vi "conexionDB.vi"() -> ()   [LabVIEW 2016]
uses:
  <vilib>/addons/database/Connection.llb/DB Tools Open Connec (Path).vi
  <vilib>/addons/database/NI_Database_API.lvlib
panel:
  out "data":variant[][](array[variant])
  out "Table Control":string[][](table)
  out "Multicolumn Listbox":i32(listbox)
  out "data 2":string[][](array[string])
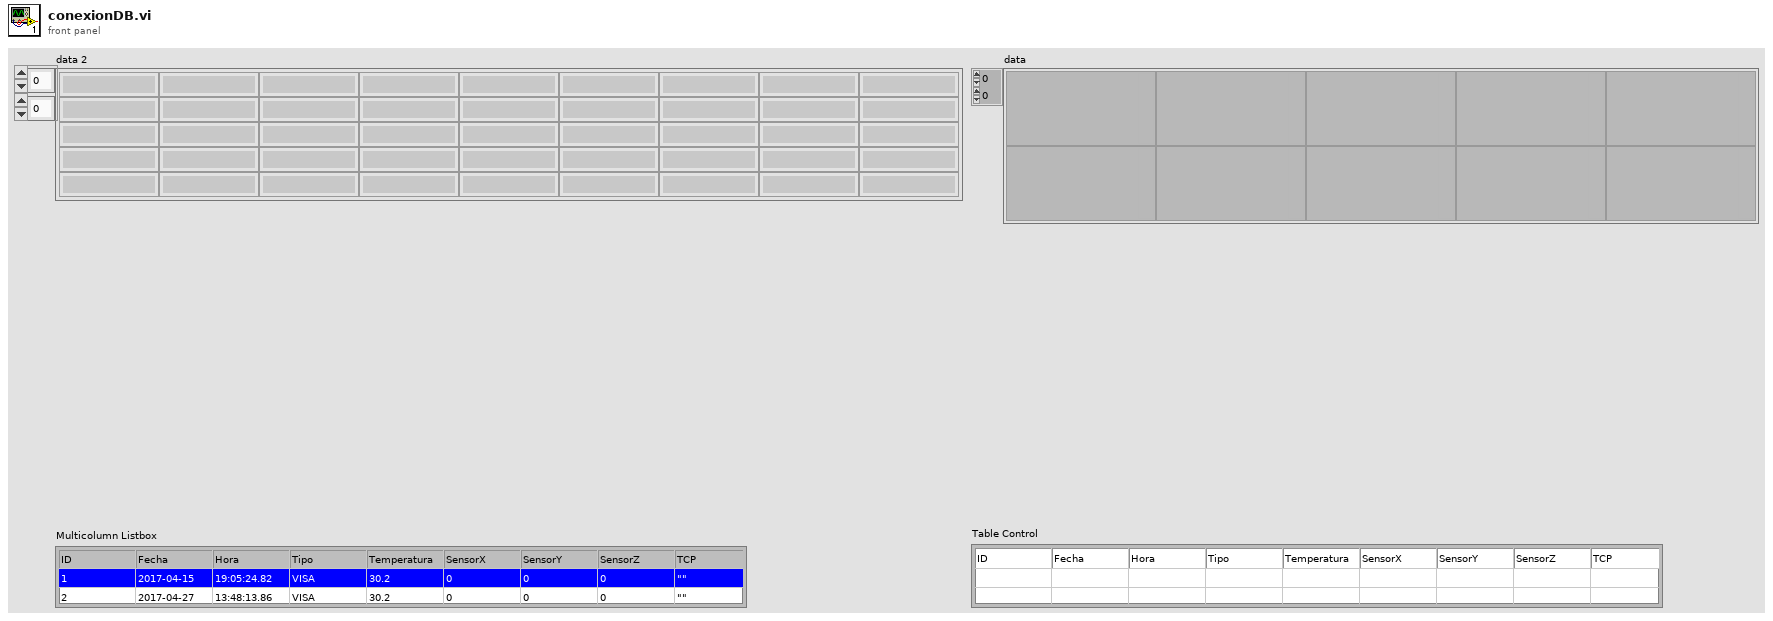
[diagram p1: front panel]
types:
  T1 = typedef "NI_Database_API.lvlib/Conn ObjectReference.ctl" = refnum<k1>
  T2 = cluster{"date/time string":string, "date/time string":string, string, dbl, dbl, dbl, dbl, string}
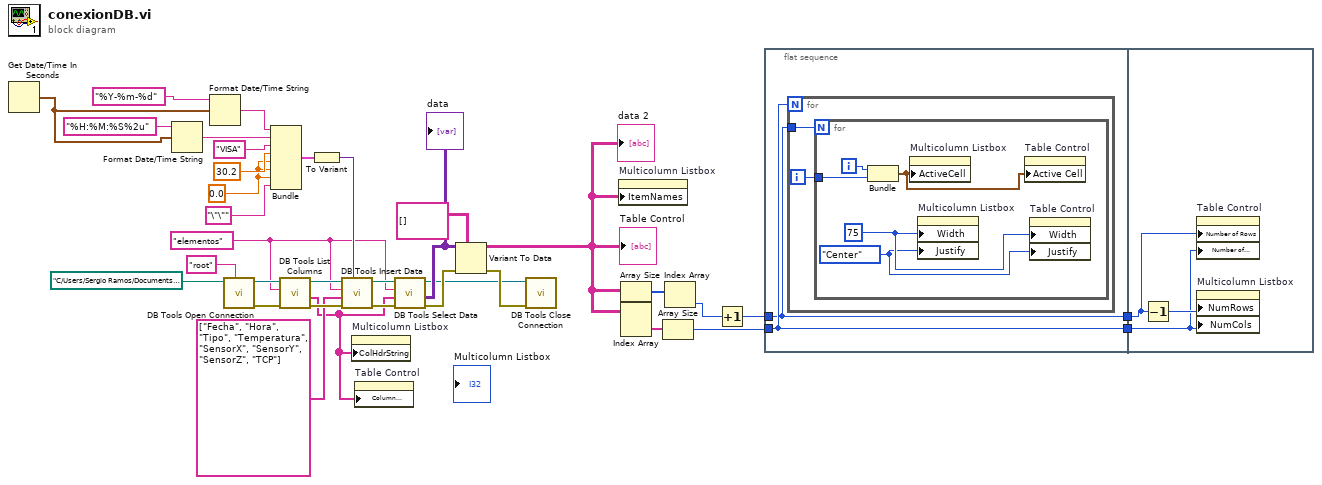
[diagram p0: block diagram]
diagram:
  w31 = 0.0
  w16 = "elementos" ("table")
  n1 = Get Date/Time In Seconds() -> (seconds since 1Jan1904=w13:timestamp)
  n2 = Format Date/Time String(time format string (%c)="%H:%M:%S%2u", seconds (now)=w13) -> (date/time string=w12:string)  [unwired: 1 in]
  n3 = Format Date/Time String(time format string (%c)="%Y-%m-%d", seconds (now)=w13) -> (date/time string=w15:string)  [unwired: 1 in]
  n4 = call-poly <vilib>:"DB Tools Open Connection.vi"("userID"="root", "connection information"=path "C:/Users/Sergio Ramos/Documents/UAQ/Desarrollo de Interfaces de Hardware II/Proyecto Original/SQLServerDB.udl") -> ("error out"=w24:errorcluster, "connection reference"=w26:T1)  [unwired: 6 in]
  n5 = Bundle("date/time string"=w15, "date/time string"=w12, "VISA", 30.2, w31, w31, w31, "\"\"") -> (w14:T2)  [unwired: 1 in]
  n6 = call <vilib>:"DB Tools List Columns.vi"("error in (no error)"=w24, "table"=w16, "connection reference"=w26) -> ("error out"=w23:errorcluster, "columns"=w1:string[], "connection reference out"=w25:T1)  [unwired: 1 in, 1 out]
  n7 = To Variant(anything=w14) -> (Variant=w28:variant)
  n8 = call <vilib>:"DB Tools Insert Data.vi"("data"=w28, "error in (no error)"=w23, "columns"=string[] ["Fecha", "Hora", "Tipo", "Temperatura", "SensorX", "SensorY", "SensorZ", "TCP"], "table"=w16, "connection reference"=w25) -> ("error out"=w27:errorcluster, "connection reference out"=w17:T1)  [unwired: 5 in]
  n9 = property on="Multicolumn Listbox" class="MCListbox (strict)"("ColHdrString"=w1) -> ()  [unwired: 2 in, 2 out]
  n10 = property on="Table Control" class="Tbl (strict)"("Column Headers[]"=w1) -> ()  [unwired: 2 in, 2 out]
  n11 = call <vilib>:"DB Tools Select Data.vi"("error in (no error)"=w27, "columns"=w1, "table"=w16, "connection reference"=w17) -> ("error out"=w20:errorcluster, "data"=w22:variant[][], "connection reference out"=w2:T1)  [unwired: 2 in]
  "data" <- w22
  n12 = Variant To Data(error in=w20, type=string[][] [], Variant=w22) -> (data=w10:string[][], error out=w19:errorcluster)
  "data 2" <- w10
  "Table Control" <- w10
  n13 = call <vilib>:"DB Tools Close Connection.vi"("error in (no error)"=w19, "connection reference"=w2) -> ()  [unwired: 5 in, 1 out]
  n14 = property on="Multicolumn Listbox" class="MCListbox (strict)"("ItemNames"=w10) -> ()  [unwired: 2 in, 2 out]
  n15 = Array Size(array=w10) -> (size(s)=w8:i32[])
  n16 = Index Array(array=w10) -> (element=w9:string[])  [unwired: 2 in]
  n17 = Array Size(array=w9) -> (size(s)=w3:i32)
  n18 = Index Array(array=w8) -> (element=w5:i32)  [unwired: 1 in]
  n19 = Increment(x=w5) -> (x+1=w4:i32)
  n20 = flat-sequence {
    tunnel: w3 -> [w37]
    tunnel: [w37] -> w7
    tunnel: w4 -> [w36]
    tunnel: [w36] -> w6
    tunnel: w7 -> [w46]
    tunnel: w6 -> [w45]
    frame #0 {
      n21 = for {
        N: w37 -> [_]
        tunnel: w36 -> [w38]
        i -> [w39]
        n22 = for {
          N: w38 -> [_]
          tunnel: w39 -> [w44]
          i -> [w43]
          w41 = enum16{"Left", "Center", "Right"}."Center" ("Active Cell:Cell Justification")
          w42 = u32 75 ("Active Cell:Cell Size:Width")
          n23 = Bundle(w43, w44) -> (w40:cluster{i32, i32})  [unwired: 1 in]
          n24 = property on="Multicolumn Listbox" class="MCListbox (strict)"("ActiveCell"=w40) -> ()  [unwired: 2 in, 2 out]
          n25 = property on="Multicolumn Listbox" class="MCListbox (strict)"("Width"=w42, "Justify"=w41) -> ()  [unwired: 2 in, 2 out]
          n26 = property on="Table Control" class="Tbl (strict)"("Active Cell"=w40) -> ()  [unwired: 2 in, 2 out]
          n27 = property on="Table Control" class="Tbl (strict)"("Width"=w42, "Justify"=w41) -> ()  [unwired: 2 in, 2 out]
        }
      }
    }
    frame #1 {
      n28 = Decrement(x=w45) -> (x-1=w47:i32)
      n29 = property on="Table Control" class="Tbl (strict)"("Number of Rows"=w45, "Number of Columns"=w46) -> ()  [unwired: 2 in, 2 out]
      n30 = property on="Multicolumn Listbox" class="MCListbox (strict)"("NumRows"=w47, "NumCols"=w46) -> ()  [unwired: 2 in, 2 out]
    }
  }
